vi "SubVI - Send Config Files.vi"(8 "error in (no error)":errorcluster, 11 "file path (use dialog)":path) -> (0 "error out":errorcluster)   [LabVIEW 2017]
panel:
  out "Remaining Files":i32
  out "x-y":dbl
  out "Timer":u32
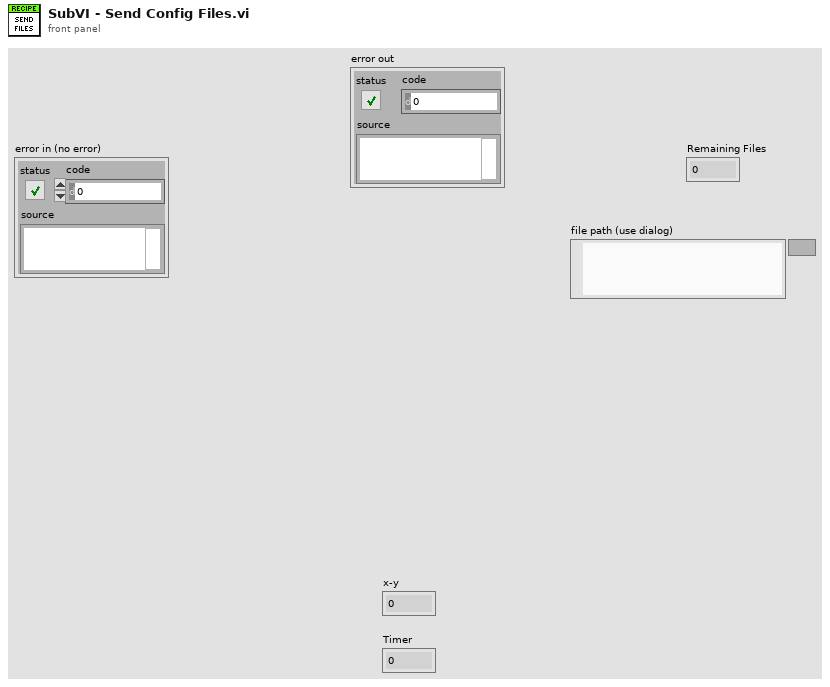
[diagram p1: front panel]
types:
  T1 = enum16{"big-endian, network order", "native, host order", "little-endian"}
  T2 = enum16{"open", "replace", "create", "open or create", "replace or create", "replace or create with confirmation"}
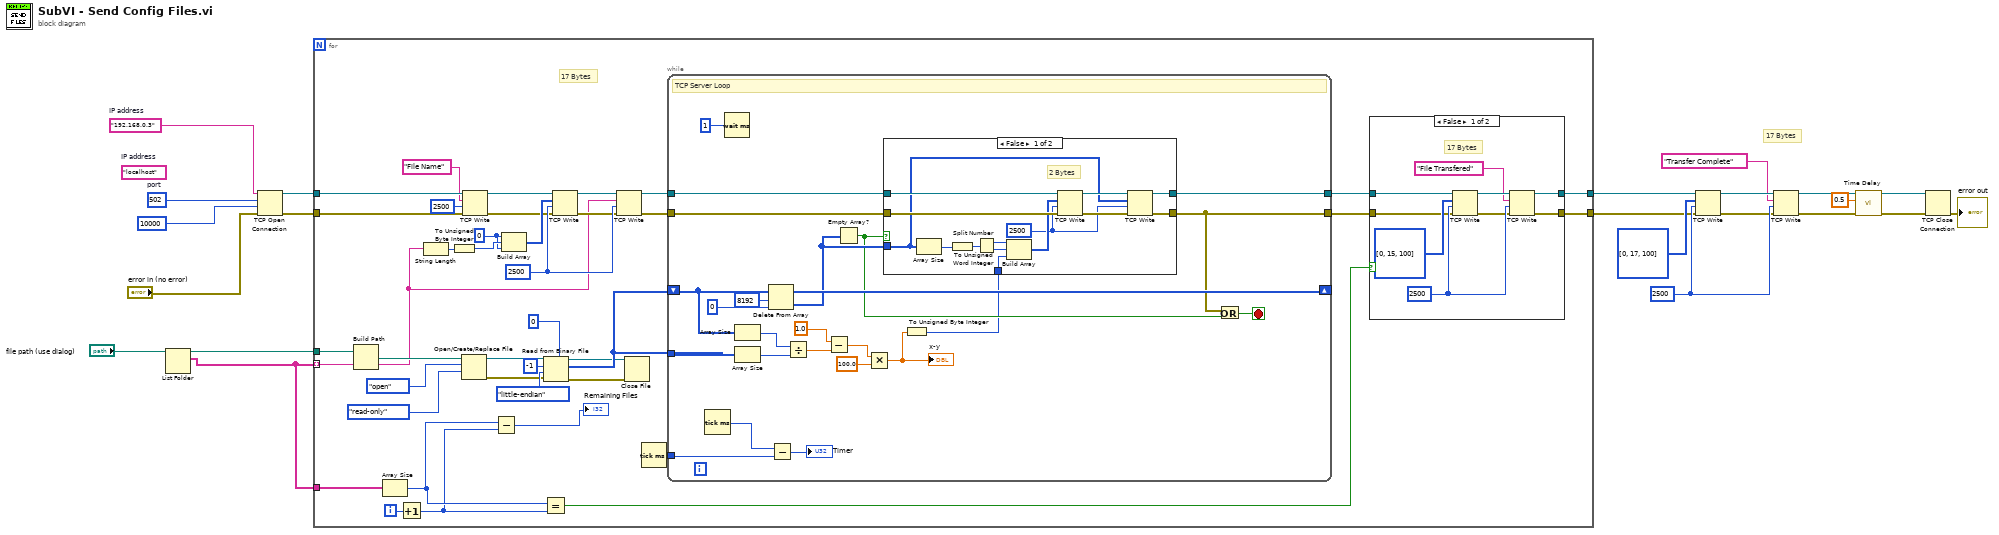
[diagram p0: block diagram]
diagram:
  w3 = "192.168.0.3"  # IP address
  w15 = 2500 ("timeout ms (25000)")
  w21 = u16 502  # port
  (unwired) "localhost"  # IP address
  # "17 Bytes"
  n1 = List Folder(path="file path (use dialog)") -> (path out=w16:path, filenames=w4:string[])  [unwired: 3 in, 2 out]
  n2 = TCP Open Connection(address=w3, remote port or service name=w21, timeout ms (60000)=10000 ("timeout ms (wait forever: -1)"), error in (no error)="error in (no error)") -> (connection ID=w19:refnum<k5>, error out=w18:errorcluster)  [unwired: 1 in]
  n3 = for {
    tunnel: w16 -> [w58]
    tunnel: w4 -> [w38] mode=indexing
    tunnel: w18 -> [w31]
    tunnel: [w44] -> w7
    tunnel: w19 -> [w33]
    tunnel: [w46] -> w8
    tunnel: w4 -> [w27]
    i -> [w26]
    w43 = 2500 ("timeout ms (25000)")
    w34 = u8 0
    # "17 Bytes"
    n4 = Build Path(base path=w58, name or relative path=w38) -> (appended path=w57:path)
    n5 = Array Size(array=w27) -> (size(s)=w24:i32)
    n6 = Increment(x=w26) -> (x+1=w23:i32)
    n7 = String Length(string=w38) -> (length=w36:i32)
    n8 = To Unsigned Byte Integer(number=w36) -> (unsigned 8bit integer=w35:u8)
    n9 = Open/Create/Replace File(file path (use dialog)=w57, operation (0:open)=T2."open", access (0:read/write)=enum16{"read/write", "read-only", "write-only"}."read-only") -> (refnum out=w53:refnum<file>, error out=w52:errorcluster)  [unwired: 3 in, 1 out]
    n10 = TCP Write(connection ID=w33, data in="File Name", error in (no error)=w31, 9:2500 ("timeout ms (25000)")) -> (connection ID out=w32:refnum<k5>, error out=w30:errorcluster)  [unwired: 1 out]
    n11 = Subtract(x=w24, y=w23) -> (x-y=→"Remaining Files":i32)
    n12 = Build Array(w34, w35, w34) -> (w37:u8[])
    n13 = Read from Binary File(5:u8 0, 8:w52, 9:T1."little-endian" ("byte order (0:big-endian, network order)"), 10:-1 ("count (1)"), 11:w53) -> (0:w49:errorcluster, 2:w51:u8[], 3:w50:refnum<file>)  [unwired: 1 in, 1 out]
    n14 = Equal?(x=w24, y=w23) -> (x = y?=w25:bool)
    n15 = TCP Write(connection ID=w32, data in=w37, error in (no error)=w30, 9:w43) -> (connection ID out=w41:refnum<k5>, error out=w42:errorcluster)  [unwired: 1 out]
    n16 = TCP Write(connection ID=w41, data in=w38, error in (no error)=w42, 9:w43) -> (connection ID out=w40:refnum<k5>, error out=w39:errorcluster)  [unwired: 1 out]
    n17 = Close File(refnum=w50, error in=w49) -> ()  [unwired: 2 out]
    n18 = Tick Count (ms)() -> (millisecond timer value=w48:u32)
    n19 = while {
      tunnel: w39 -> [w87]
      tunnel: w40 -> [w88]
      tunnel: [w94] -> w47
      tunnel: [w89] -> w45
      shift-right: [w91] -> _
      shift-left: w51 -> [w83]
      tunnel: w51 -> [w84]
      tunnel: w48 -> [w75]
      stop <- w90 stop-if-true
      # "TCP Server Loop"
      n20 = Tick Count (ms)() -> (millisecond timer value=w76:u32)
      n21 = Wait (ms)(milliseconds to wait=u32 1) -> ()  [unwired: 1 out]
      n22 = Array Size(array=w83) -> (size(s)=w81:i32)
      n23 = Array Size(array=w84) -> (size(s)=w82:i32)
      n24 = Delete From Array(array=w83, length=8192, index=0) -> (deleted portion=w86:u8[], array with subset deleted=w91:u8[])
      n25 = Subtract(x=w76, y=w75) -> (x-y=→"Timer":u32)
      n26 = Divide(x=w81, y=w82) -> (x/y=w79:dbl)
      n27 = Subtract(x=1.0, y=w79) -> (x-y=w78:dbl)
      n28 = Empty Array?(array=w86) -> (empty?=w85:bool)
      n29 = Multiply(x=w78, y=100.0) -> (x*y=w73:dbl)
      "x-y" <- w73
      n30 = To Unsigned Byte Integer(number=w73) -> (unsigned 8bit integer=w72:u8)
      n31 = case shown="False" w85 {
        tunnel: [w109 w111] -> w94
        tunnel: [w108 w110] -> w89
        tunnel: w88 -> [w107 w111]
        tunnel: w87 -> [w105 w110]
        tunnel: w86 -> [w103 _]
        tunnel: w72 -> [w96 _]
        frame False {
          w97 = 2500 ("timeout ms (25000)")
          # "2 Bytes"
          n32 = Array Size(array=w103) -> (size(s)=w102:i32)
          n33 = To Unsigned Word Integer(number=w102) -> (unsigned 16bit integer=w101:u16)
          n34 = Split Number(x=w101) -> (hi(x)=w100:u8, lo(x)=w99:u8)
          n35 = Build Array(w100, w99, w96) -> (w98:u8[])
          n36 = TCP Write(connection ID=w107, data in=w98, error in (no error)=w105, 9:w97) -> (connection ID out=w106:refnum<k5>, error out=w104:errorcluster)  [unwired: 1 out]
          n37 = TCP Write(connection ID=w106, data in=w103, error in (no error)=w104, 9:w97) -> (connection ID out=w109:refnum<k5>, error out=w108:errorcluster)  [unwired: 1 out]
        }
        frame True {
        }
      }
      n38 = Or(x=w89, y=w85) -> (x .or. y?=w90:bool)
    }
    n39 = case shown="False" w25 {
      tunnel: w47 -> [w64 w71]
      tunnel: [w63 w71] -> w46
      tunnel: w45 -> [w62 w70]
      tunnel: [w61 w70] -> w44
      frame False {
        w69 = 2500 ("timeout ms (25000)")
        # "17 Bytes"
        n40 = TCP Write(connection ID=w64, data in=u8[] [0, 15, 100], error in (no error)=w62, 9:w69) -> (connection ID out=w67:refnum<k5>, error out=w68:errorcluster)  [unwired: 1 out]
        n41 = TCP Write(connection ID=w67, data in="File Transfered", error in (no error)=w68, 9:w69) -> (connection ID out=w63:refnum<k5>, error out=w61:errorcluster)  [unwired: 1 out]
      }
      frame True {
      }
    }
  }
  n42 = TCP Write(connection ID=w8, data in=u8[] [0, 17, 100], error in (no error)=w7, 9:w15) -> (connection ID out=w13:refnum<k5>, error out=w14:errorcluster)  [unwired: 1 out]
  n43 = TCP Write(connection ID=w13, data in="Transfer Complete", error in (no error)=w14, 9:w15) -> (connection ID out=w6:refnum<k5>, error out=w11:errorcluster)  [unwired: 1 out]
  n44 = call "Time Delay"("error in (no error)"=w11, "Delay Time (s)"=0.5) -> ("error out"=w5:errorcluster)  [unwired: 9 in]
  n45 = TCP Close Connection(connection ID=w6, error in (no error)=w5) -> (error out=→"error out":errorcluster)  [unwired: 1 in, 1 out]
